vi "sub_2x8MAT.vi"(6 "V":dbl, 9 "U":dbl, 10 "Y":dbl, 11 "X":dbl) -> (3 "Real Matrix":T1)   [LabVIEW 2020]
uses:
  <vilib>/Analysis/Matrix/Datatypes/RealMatrix.ctl
  <vilib>/Analysis/Matrix/Numeric/Conversions/Array To Matrix - RA.vi
  <vilib>/Analysis/Matrix/NI_Matrix.lvlib
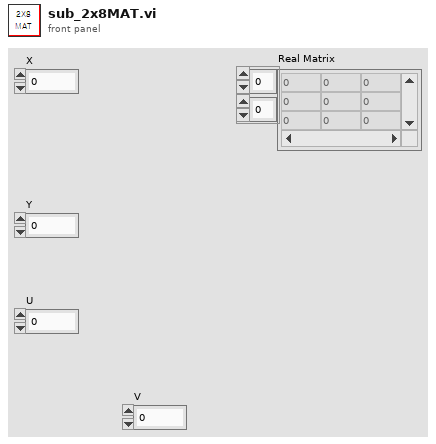
[diagram p1: front panel]
types:
  T1 = typedef "NI_Matrix.lvlib/RealMatrix.ctl" = dbl[][]
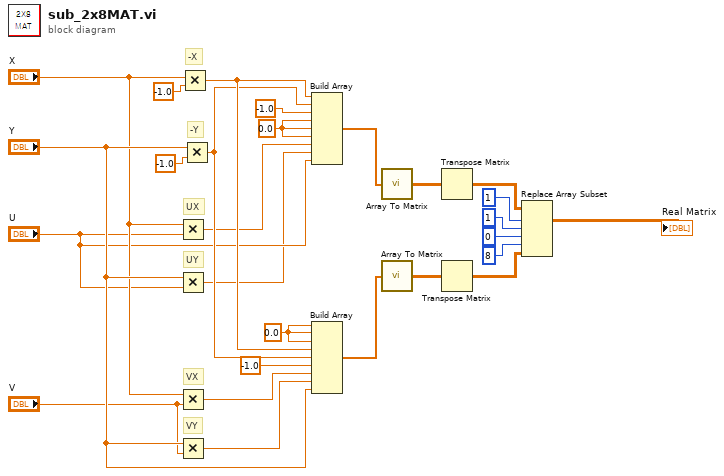
[diagram p0: block diagram]
diagram:
  w8 = 0.0 ("원소")
  w4 = 0.0 ("원소")
  # "VY"
  # "VX"
  # "UY"
  # "UX"
  # "-Y"
  # "-X"
  n1 = Multiply(x="X", y="U") -> (x*y=w5:dbl)
  n2 = Multiply(x="Y", y="U") -> (x*y=w6:dbl)
  n3 = Multiply(x="X", y="V") -> (x*y=w12:dbl)
  n4 = Multiply(x="Y", y="V") -> (x*y=w13:dbl)
  n5 = Multiply(x="X", y=-1.0) -> (x*y=w10:dbl)
  n6 = Multiply(x="Y", y=-1.0) -> (x*y=w9:dbl)
  n7 = Build Array(w10, w9, -1.0 ("원소"), w4, w4, w4, w5, w6, "U") -> (w17:dbl[])
  n8 = Build Array(w8, w8, w8, w10, w9, -1.0 ("원소"), w12, w13, "Y") -> (w18:dbl[])
  n9 = call-poly <vilib>:"Array To Matrix.vi"("Real 1D Array"=w17) -> ("Real Matrix (Column Vector)"=w19:T1)
  n10 = call-poly <vilib>:"Array To Matrix.vi"("Real 1D Array"=w18) -> ("Real Matrix (Column Vector)"=w20:T1)
  n11 = Transpose Matrix(1:w19) -> (0:w21:T1)
  n12 = Transpose Matrix(1:w20) -> (0:w22:T1)
  n13 = Replace Array Subset(array=w21, new element=w22, index (dim 0)=1 ("행 1"), index (dim 1)=1 ("행 N"), index (dim 2)=0 ("열 1"), index (dim 3)=8 ("열 N")) -> (→"Real Matrix":T1)
